vi "Open_USB.vi"(8 "entrée d'erreur (pas d'erreur)":errorcluster, 9 "Timeout de VISA Open (0)":u32, 10 "Access Mode":T1 items=["VISA Defaults"=0, "Exclusive Lock"=1, "Load Configured Settings"=4], 11 "Nom de ressource VISA":refnum<visa-resource-name>) -> (0 "error out":errorcluster, 3 "Nom de ressource VISA ouverte":refnum<visa-resource-name>)   [LabVIEW 2013]
uses:
  <vilib>/Instr/_visa.llb/VISA Open Access Mode.ctl
  <vilib>/Instr/_visa.llb/Select Event Type.ctl
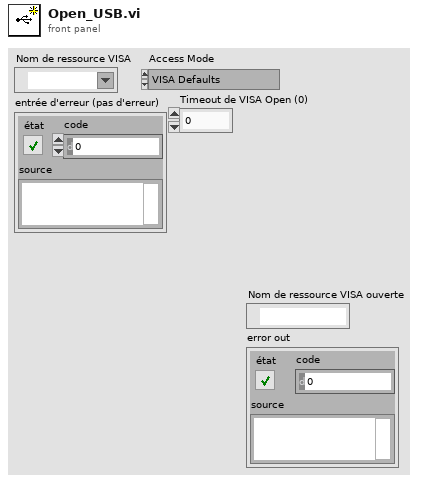
[diagram p1: front panel]
types:
  T1 = typedef "VISA Open Access Mode.ctl" = u32
  T2 = typedef "Select Event Type.ctl" = u32
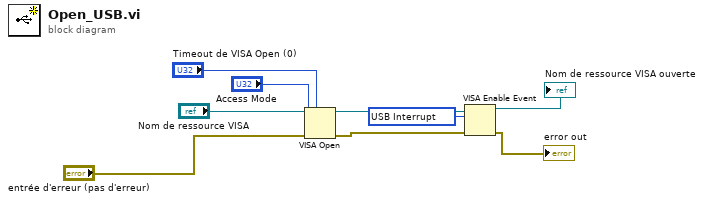
[diagram p0: block diagram]
diagram:
  w7 = T2 1073684535 items=["Service Request"=1073684491, "Trigger"=3221168138, "Clear"=1073684493, "VXI Signal"=1073684512, "VXI/VME Interrupt"=3221168161, "VXI/VME Sysfail"=1073684509, "VXI/VME Sysreset"=1073684510, "GPIB-CIC"=1073684498, "GPIB-Talk"=1073684499, "GPIB-Listen"=1073684500, "PXI Interrupt"=1073684514, "Serial Break"=1073684515, "Serial TermChar"=1073684516, "Serial CTS"=1073684521, "Serial DSR"=1073684522, "Serial DCD"=1073684524, "Serial RI"=1073684526, "Serial Character"=1073684533, "USB Interrupt"=1073684535, "All Enabled"=1073709055] ("Event Type")
  n1 = VISA Open(timeout (0)="Timeout de VISA Open (0)", access mode="Access Mode", error in (no error)="entrée d'erreur (pas d'erreur)", VISA resource name="Nom de ressource VISA") -> (VISA resource name=w9:refnum<visa-resource-name>, error out=w8:errorcluster)  [unwired: 1 in]
  n2 = VISA Enable Event(8:w8, 10:w7, 11:w9) -> (0:→"error out":errorcluster, 3:→"Nom de ressource VISA ouverte":refnum<visa-resource-name>)  [unwired: 1 in]
